vi "Query Harmonics Order Size.vi"(8 "error in (no error)":errorcluster, 11 "VISA resource name":refnum<visa-resource-name>) -> (0 "error out":errorcluster, 2 "Number of Harmonics Order":i32, 3 "VISA resource name out":refnum<visa-resource-name>)   [LabVIEW 2018, in "Yokogawa WT300 Series.lvlib"]
doc: "Queries the number of output harmonic order of the harmonic measurement numeric list data."
uses:
  Yokogawa WT300 Series.lvlib
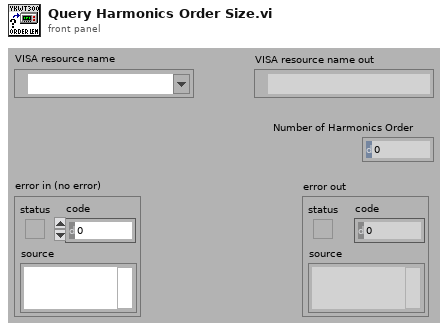
[diagram p1: front panel]
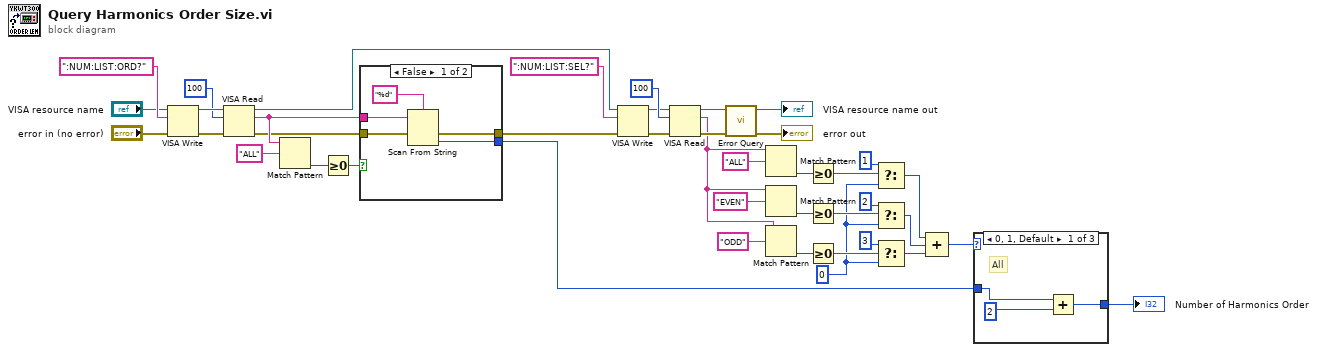
[diagram p0: block diagram]
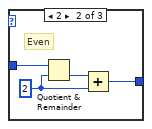
[diagram p2: hidden frame]
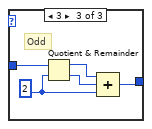
[diagram p3: hidden frame]
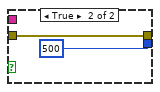
[diagram p4: hidden frame]
diagram:
  w7 = 0 ("t")
  n1 = VISA Write ("VISA書き込み")(VISA resource name="VISA resource name", write buffer=":NUM:LIST:ORD?", error in (no error)="error in (no error)") -> (VISA resource name out=w40:refnum<visa-resource-name>, error out=w41:errorcluster)  [unwired: 1 out]
  n2 = VISA Read ("VISA読み取り")(VISA resource name=w40, byte count=u32 100, error in (no error)=w41) -> (VISA resource name out=w29:refnum<visa-resource-name>, read buffer=w25:string, error out=w24:errorcluster)  [unwired: 1 out]
  n3 = Match Pattern(string=w25, regular expression="ALL") -> (offset past match=w27:i32)  [unwired: 1 in, 3 out]
  n4 = Greater Or Equal To 0?(x=w27) -> (x >= 0?=w26:bool)
  n5 = case shown="False" w26 {
    tunnel: w25 -> [w42 _]
    tunnel: w24 -> [w45 w47]
    tunnel: [w44 500] -> w1
    tunnel: [w43 w47] -> w23
    frame False {
      n6 = Scan From String ("文字列からスキャン")(format string="%d", input string=w42, error in=w45) -> (error out=w43:errorcluster, output 1=w44:i32)  [unwired: 2 in, 2 out]
    }
    frame True {
    }
  }
  n7 = VISA Write ("VISA書き込み")(VISA resource name=w29, write buffer=":NUM:LIST:SEL?", error in (no error)=w23) -> (VISA resource name out=w32:refnum<visa-resource-name>, error out=w31:errorcluster)  [unwired: 1 out]
  n8 = VISA Read ("VISA読み取り")(VISA resource name=w32, byte count=u32 100, error in (no error)=w31) -> (VISA resource name out=w21:refnum<visa-resource-name>, read buffer=w2:string, error out=w20:errorcluster)  [unwired: 1 out]
  n9 = call "Error Query.vi"("error in (no error)"=w20, "VISA resource name"=w21) -> ("error out"=→"error out":errorcluster, "VISA resource name out"=→"VISA resource name out":refnum<visa-resource-name>)  [unwired: 6 in, 2 out]
  n10 = Match Pattern(string=w2, regular expression="ALL") -> (offset past match=w22:i32)  [unwired: 1 in, 3 out]
  n11 = Match Pattern(string=w2, regular expression="EVEN") -> (offset past match=w18:i32)  [unwired: 1 in, 3 out]
  n12 = Match Pattern(string=w2, regular expression="ODD") -> (offset past match=w15:i32)  [unwired: 1 in, 3 out]
  n13 = Greater Or Equal To 0?(x=w22) -> (x >= 0?=w13:bool)
  n14 = Greater Or Equal To 0?(x=w18) -> (x >= 0?=w9:bool)
  n15 = Greater Or Equal To 0?(x=w15) -> (x >= 0?=w8:bool)
  n16 = Select(t=1, s=w13, f=w7) -> (s? t:f=w6:i32)
  n17 = Select(t=2, s=w9, f=w7) -> (s? t:f=w4:i32)
  n18 = Select(t=3, s=w8, f=w7) -> (s? t:f=w5:i32)
  n19 = Compound Arithmetic op=ADD(w6, w4, w5) -> (w3:i32)
  n20 = case shown="0, 1, Default" w3 {
    tunnel: w1 -> [w49 w52 w56]
    tunnel: [w51 w53 w60] -> w19
    frame 0, 1, Default {
      # "All"
      n21 = Add(x=w49, y=2) -> (x+y=w51:i32)
    }
    frame 2 {
      w54 = 2 ("y")
      # "Even"
      n22 = Quotient & Remainder(x=w52, y=w54) -> (floor(x/y)=w55:i32)  [unwired: 1 out]
      n23 = Add(x=w55, y=w54) -> (x+y=w53:i32)
    }
    frame 3 {
      w57 = 2 ("y")
      # "Odd"
      n24 = Quotient & Remainder(x=w56, y=w57) -> (x-y*floor(x/y)=w59:i32, floor(x/y)=w58:i32)
      n25 = Compound Arithmetic op=ADD(w59, w58, w57) -> (w60:i32)
    }
  }
  "Number of Harmonics Order" <- w19
